vi "LatLonConverter.vi"(10 "lon (GPS string)":string, 11 "lat (GPS string)":string) -> (2 "lon (degrees)":dbl, 3 "lat (degrees)":dbl)   [LabVIEW 2019]
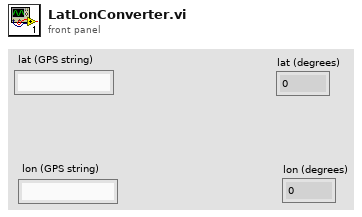
[diagram p1: front panel]
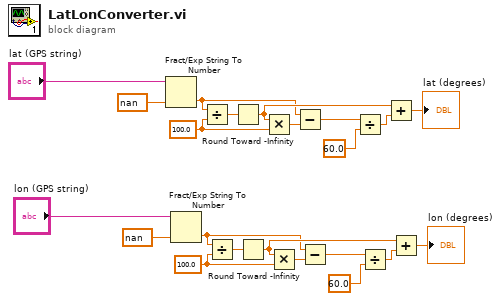
[diagram p0: block diagram]
diagram:
  w9 = 100.0 ("y")
  w20 = 100.0 ("y")
  n1 = Fract/Exp String To Number(string="lat (GPS string)", default (0 dbl)=nan) -> (number=w14:dbl)  [unwired: 2 in, 1 out]
  n2 = Fract/Exp String To Number(string="lon (GPS string)", default (0 dbl)=nan) -> (number=w3:dbl)  [unwired: 2 in, 1 out]
  n3 = Divide(x=w14, y=w20) -> (x/y=w21:dbl)
  n4 = Divide(x=w3, y=w9) -> (x/y=w10:dbl)
  n5 = Round Toward -Infinity(1:w21) -> (0:w16:dbl)
  n6 = Round Toward -Infinity(1:w10) -> (0:w5:dbl)
  n7 = Multiply(x=w16, y=w20) -> (x*y=w19:dbl)
  n8 = Multiply(x=w5, y=w9) -> (x*y=w8:dbl)
  n9 = Subtract(x=w14, y=w19) -> (x-y=w17:dbl)
  n10 = Subtract(x=w3, y=w8) -> (x-y=w6:dbl)
  n11 = Divide(x=w17, y=60.0) -> (x/y=w15:dbl)
  n12 = Divide(x=w6, y=60.0) -> (x/y=w4:dbl)
  n13 = Add(x=w16, y=w15) -> (x+y=→"lat (degrees)":dbl)
  n14 = Add(x=w5, y=w4) -> (x+y=→"lon (degrees)":dbl)
